vi "RadpsToRPM.vi"(1 "radps":dbl) -> (0 "rpm":dbl)   [LabVIEW 2018]
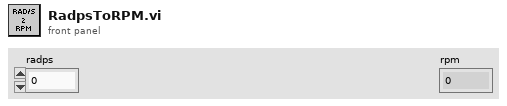
[diagram p1: front panel]
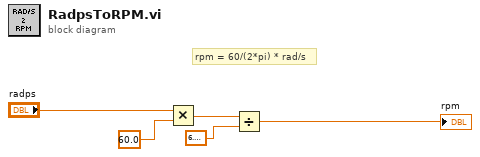
[diagram p0: block diagram]
diagram:
  # "rpm = 60/(2*pi) * rad/s"
  n1 = Multiply(x="radps", y=60.0) -> (x*y=w3:dbl)
  n2 = Divide(x=w3, y=6.283185307179586) -> (x/y=→"rpm":dbl)
